vi "SVT Dynamic Range (Time) (1 Ch).vi"(0 "scaled signal [EU]":waveform(dbl), 2 "frequency range":T10={"start frequency"=-1.0, "stop frequency"=-1.0} {"stop frequency" format="%.2f"; "start frequency" format="%.2f"}, 3 "advanced span [Hz]":dbl=-1.0 format="%.2f", 5 "error in (no error)":errorcluster, 6 "desired units":T9={"dynamic range units"=enum."dB", "detected fundamental amplitude units"=enum."EU peak"}, 7 "full scale amplitude [EU peak]":dbl=10.0 format="%.2f", 9 "expected fundamental\nfrequency [Hz]":dbl=-1.0 format="%.2f") -> (11 "detected fundamental\nfrequency [Hz]":dbl=nan format="%.2f", 12 "unit labels":T8, 13 "detected fundamental\namplitude":dbl=nan format="%.2f", 14 "complex spectrum":T7={"complex spectrum response"={"f0"=0.0, "df"=1.0, "complex spectrum"=[]}, "spectrum info"={"channel name"="", "description"="", "x-axis units"=0, "spectral info"={"spectrum type"=enum."Power [Magnitude^2]", "linear/dB"=enum."linear", "window"=0, "window size"=0, "FFT size"=0}, "engineering units"=0, "custom label"="", "dB reference [EU]"=0.0, "peak units"=enum."rms", "weighting filter"=0, "spectral density?"=FALSE, "unit label"="", "spectrum skewed?"=FALSE, "complimentary spectrum units"=enum."none"}} {"spectrum info"."x-axis units" items=["Time (s)"=0, "Frequency-CB (Hz)"=1, "Frequency-CPB (Hz)"=1248, "Frequency-Arbitrary (Hz)"=2357, "Quefrency (s)"=2, "Revolutions (rev)"=3, "Order"=4, "Speed (RPM)"=11, "Speed (rad/s)"=21, "Index"=65535]; "spectrum info"."weighting filter" items=["Linear", "A-weighting", "B-weighting", "C-weighting", "ITU-R 468-4", "Dolby", "CCITT", "C-message", "Wb", "Wc", "Wd", "We", "Wf", "Wh", "Wj", "Wk", "Wm", "AES17 20 kHz lowpass", "AES17 40 kHz lowpass", "AES17 20 kHz highpass", "AES17 40 kHz highpass"]; "spectrum info"."dB reference [EU]" format="%.2f"; "spectrum info"."engineering units" items=["custom..."=0, "V"=1, "A"=21, "C"=30, "pC"=31, "s"=32, "-"=29, "Pa"=2, "N"=20, "g"=3, "m/s^2"=4, "m/s"=5, "m"=6, "mm/s"=12, "mm"=13, "micron/s"=14, "micron"=15, "in/s^2"=7, "in/s"=8, "in"=9, "mil/s"=10, "mil"=11, "rad/s^2"=16, "rad/s"=17, "rad"=18, "deg/s^2"=26, "deg/s"=27, "deg"=28, "RPM"=22, "cycle/s^2"=23, "Hz"=24, "cycle"=25, "strain"=19]; "spectrum info"."spectral info"."window" items=["None "=0, "Hanning"=1, "Hamming"=2, "Blackman-Harris"=3, "Exact Blackman"=4, "Blackman"=5, "Flat Top"=6, "4 Term B-Harris "=7, "7 Term B-Harris"=8, "Low Sidelobe"=9, "Force - Exponential"=10, "Gaussian"=62]; "complex spectrum response"."complex spectrum" format="%.2f"; "complex spectrum response"."df" format="%.2f"; "complex spectrum response"."f0" format="%.2f"}, 16 "dynamic range":dbl=nan format="%.2f", 19 "error out":errorcluster)   [LabVIEW 2017, in "SoundVib_SingleTone.lvlib"]
doc: "Computes the dynamic range of a channel based on<B> scaled signal</B> and <B>full scale amplitude</B> and returns the detected fundamental frequency, detected fundamental amplitude, and dynamic range. This VI does not maintain state internally; you can use this VI in a loop to process multiple blocks. Wire data to the <B>scaled signal [EU]</B> input to determine the polymorphic instance to use or manually select the instance."
uses:
  <vilib>/addons/Sound and Vibration/svt_Single Tone Measurements/SoundVib_SingleTone.lvlib
  <vilib>/addons/_NISVFA/_Shared subVIs/Controls/svc_Spectrum Info.ctl
  <vilib>/addons/_NISVFA/_Shared subVIs/Controls/svc_X-Axis Units.ctl
  <vilib>/addons/_NISVFA/_Shared subVIs/Controls/svc_Spectrum Type.ctl
  <vilib>/addons/_NISVFA/_Shared subVIs/Controls/svc_Engineering Units Text Ring.ctl
  <vilib>/addons/_NISVFA/_Shared subVIs/Controls/svc_Weighting Filter Text Ring.ctl
  <vilib>/addons/_NISVFA/_Shared subVIs/Controls/svc_Complimentary Spectrum Units.ctl
  <vilib>/addons/_NISVFA/_Shared subVIs/Controls/svc_Window.ctl
  <vilib>/addons/Sound and Vibration/svt_Distortion/SoundVib_Distortion.lvlib
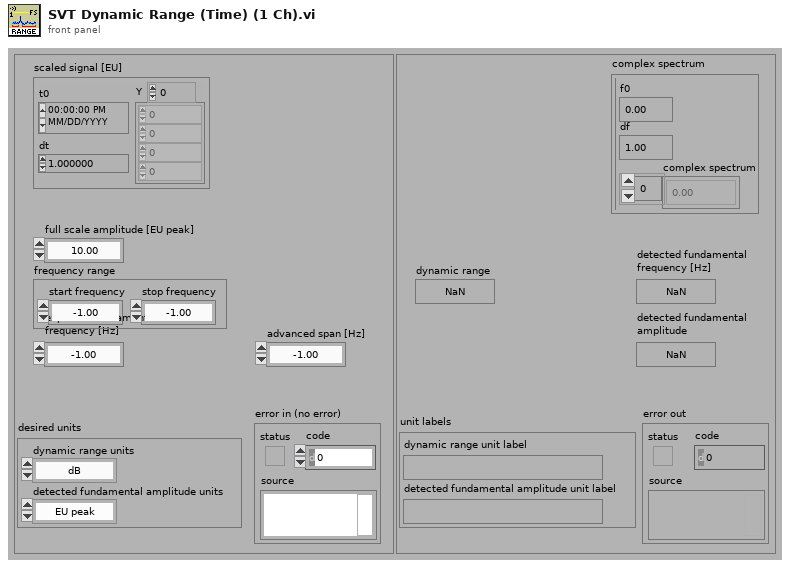
[diagram p1: front panel]
types:
  T1 = typedef "svc_Spectrum Info.ctl" = cluster{"channel name":string, "description":string, "x-axis units":T2, "spectral info":cluster{"spectrum type":T3, "linear/dB":enum16{"linear", "dB"}, "window":u16, "window size":i32, "FFT size":i32}, "engineering units":T4, "custom label":string, "dB reference [EU]":dbl, "peak units":enum16{"rms", "peak", "peak-peak"}, "weighting filter":T5, "spectral density?":bool, "unit label":string, "spectrum skewed?":bool, "complimentary spectrum units":T6}
  T2 = typedef "svc_X-Axis Units.ctl" = u16
  T3 = typedef "svc_Spectrum Type.ctl" = enum16{"FFT Spectrum [complex]", "Amplitude [Magnitude]", "Power [Magnitude^2]", "Cross Spectrum [complex]", "Frequency Response [Complex]"}
  T4 = typedef "svc_Engineering Units Text Ring.ctl" = u16
  T5 = typedef "svc_Weighting Filter Text Ring.ctl" = u16
  T6 = typedef "svc_Complimentary Spectrum Units.ctl" = enum16{"none", "radians", "degrees", "cycles", "imaginary"}
  T7 = cluster{"complex spectrum response":cluster{"f0":dbl, "df":dbl, "complex spectrum":cdb[]}, "spectrum info":T1}
  T8 = cluster{"dynamic range unit label":string, "detected fundamental amplitude unit label":string}
  T9 = cluster{"dynamic range units":enum16{"dB", "ENOB"}, "detected fundamental amplitude units":enum16{"EU rms", "EU peak", "EU peak-peak"}}
  T10 = cluster{"start frequency":dbl, "stop frequency":dbl}
  T11 = cluster{"dynamic range unit label":string, "fundamental amplitude unit label":string}
  T12 = typedef "svc_Window.ctl" = u32
  T13 = cluster{"complex spectrum":cluster{"f0":dbl, "df":dbl, "complex spectrum":cdb[]}, "spectrum info":T1}
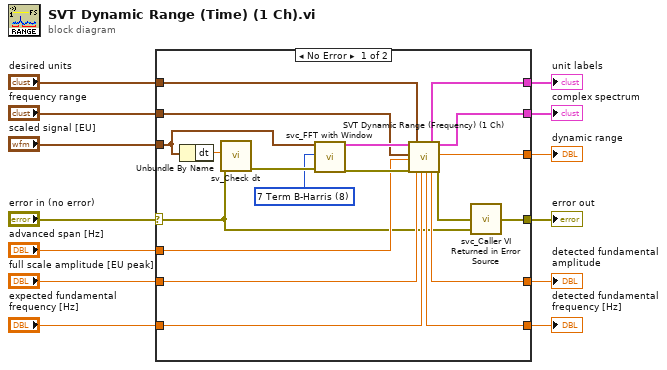
[diagram p0: block diagram]
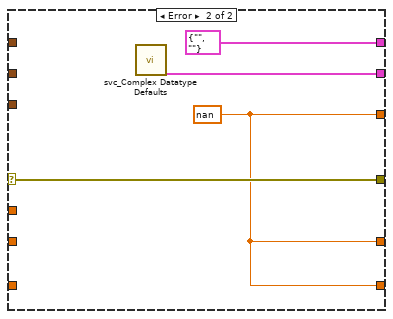
[diagram p2: hidden frame]
diagram:
  n1 = case shown="No Error" "error in (no error)" {
    selector: "error in (no error)" -> [w14 w36]
    tunnel: [w30 w33] -> w2
    tunnel: [w20 w36] -> w13
    tunnel: "scaled signal [EU]" -> [w15 _]
    tunnel: "expected fundamental\nfrequency [Hz]" -> [w28 _]
    tunnel: "full scale amplitude [EU peak]" -> [w27 _]
    tunnel: "frequency range" -> [w25 _]
    tunnel: "desired units" -> [w24 _]
    tunnel: [w26 T11 {"dynamic range unit label"="", "fundamental amplitude unit label"=""} ("unit labels")] -> w6
    tunnel: [w23 w35] -> w5
    tunnel: [w22 w35] -> w4
    tunnel: [w21 w35] -> w3
    tunnel: "advanced span [Hz]" -> [w17 _]
    frame No Error {
      w18 = T12 8 items=["None ", "Hanning", "Hamming", "Blackman-Harris", "Exact Blackman", "Blackman", "Flat Top", "4 Term B-Harris ", "7 Term B-Harris", "Low Sidelobe"] ("window")
      n2 = Unbundle By Name(w15) -> ("dt"=w16:dbl)
      n3 = call <vilib>:"sv_Check dt.vi"("error in"=w14, "dt"=w16) -> ("error out"=w19:errorcluster)  [unwired: 8 in, 1 out]
      n4 = call <vilib>:"svc_FFT with Window.vi"("time signal in [EU]"=w15, "window"=w18, "error in (no error)"=w19) -> ("complex spectrum"=w32:T7, "error out"=w31:errorcluster)  [unwired: 15 in]
      n5 = call <vilib>:"SVT Dynamic Range (Frequency) (1 Ch).vi"("complex spectrum"=w32, "frequency range"=w25, "advanced span [Hz]"=w17, "error in (no error)"=w31, "desired units"=w24, "full scale amplitude [EU peak]"=w27, "expected fundamental\nfrequency [Hz]"=w28) -> ("detected fundamental\nfrequency [Hz]"=w23:dbl, "unit labels"=w26:T8, "detected fundamental\namplitude"=w22:dbl, "dup complex spectrum"=w30:T7, "dynamic range"=w21:dbl, "error out"=w29:errorcluster)  [unwired: 7 in]
      n6 = call <vilib>:"svc_Caller VI Returned in Error Source.vi"("warning input to caller"=w14, "error in (no error)"=w29) -> ("error out"=w20:errorcluster)  [unwired: 3 in]
    }
    frame Error {
      w35 = nan
      n7 = call <vilib>:"svc_Complex Datatype Defaults.vi"() -> ("complex spectrum"=w33:T13)  [unwired: 11 in, 8 out]
    }
  }
  "error out" <- w13
  "dynamic range" <- w3
  "unit labels" <- w6
  "detected fundamental\namplitude" <- w4
  "detected fundamental\nfrequency [Hz]" <- w5
  "complex spectrum" <- w2
